vi "Initialize.vi"(7 "Serial Configuration":T1={"Baud Rate"=9600, "Flow Control"=0, "Parity"=0, "Data Bits"=8} {"Flow Control" items=["NONE", "SOFTWARE"]; "Data Bits" items=["7"=7, "8"=8]; "Parity" items=["NONE", "ODD", "EVEN"]; "Baud Rate" items=["300"=300, "600"=600, "1200"=1200, "2400"=2400, "4800"=4800, "9600"=9600, "19200"=19200]}, 8 "error in (no error)":errorcluster, 9 "Reset (True)":bool=TRUE, 10 "ID Query (True)":bool=TRUE, 11 "VISA resource name":refnum<visa-resource-name>) -> (0 "error out":errorcluster, 3 "VISA resource name out":refnum<visa-resource-name>)   [LabVIEW 2025, in "Chroma 19052.lvlib"]
doc: "Establishes communication with the instrument and optionally performs an instrument identification query and/or an instrument reset. It also places the instrument in a default state needed for other instrument driver operations. Therefore, call this VI before calling other instrument driver VIs for this instrument. Generally, you need to call the <b>Initialize</b> VI only once at the beginning of an application."
uses:
  <instrlib>/Chroma 19052/Chroma 19052.lvlib
  <vilib>/ErrorRing/Error Ring.xnode
panel:
  # "(c) 2025 RAMON TABOADA.  ALL RIGHTS RESERVED."
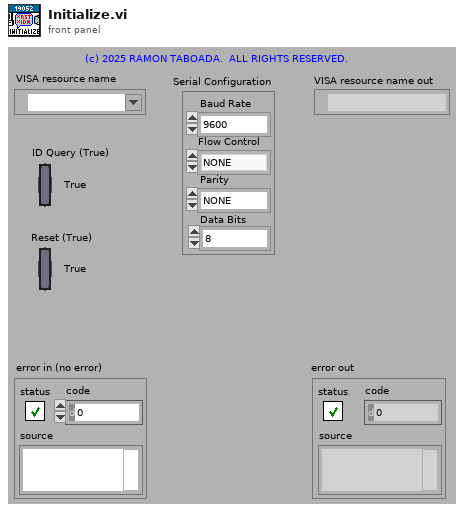
[diagram p1: front panel]
types:
  T1 = cluster{"Baud Rate":u32, "Flow Control":u16, "Parity":u16, "Data Bits":u16}
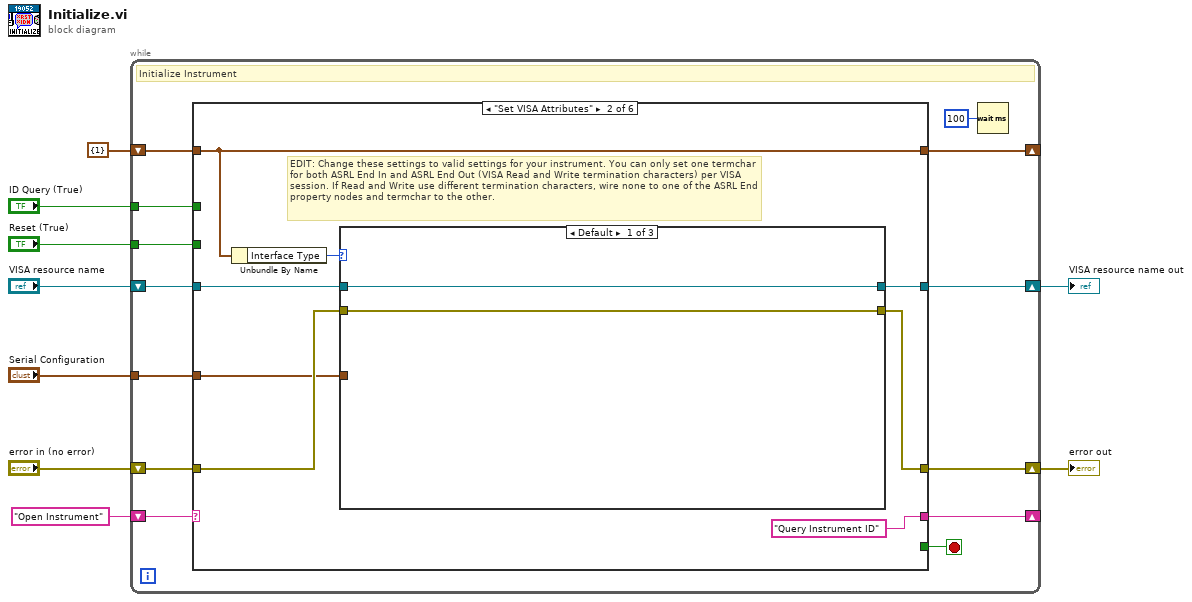
[diagram p0: block diagram]
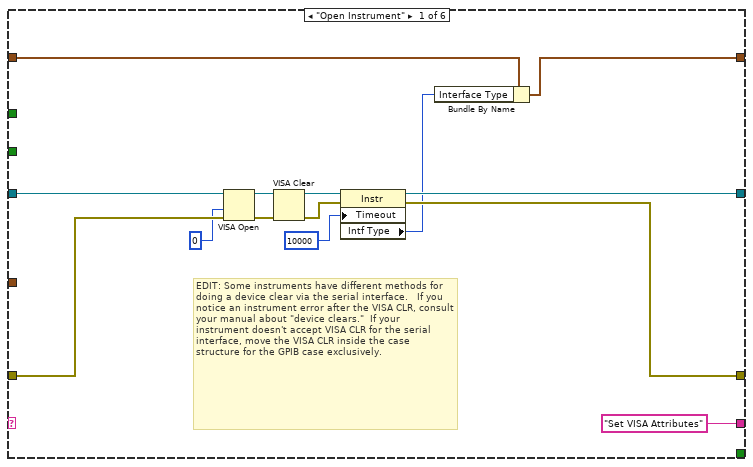
[diagram p2: hidden frame]
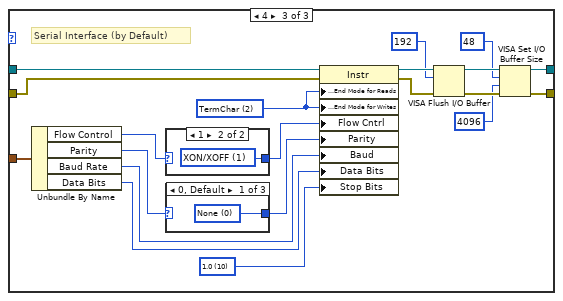
[diagram p4: hidden frame]
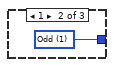
[diagram p5: hidden frame]
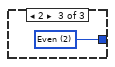
[diagram p6: hidden frame]
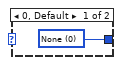
[diagram p7: hidden frame]
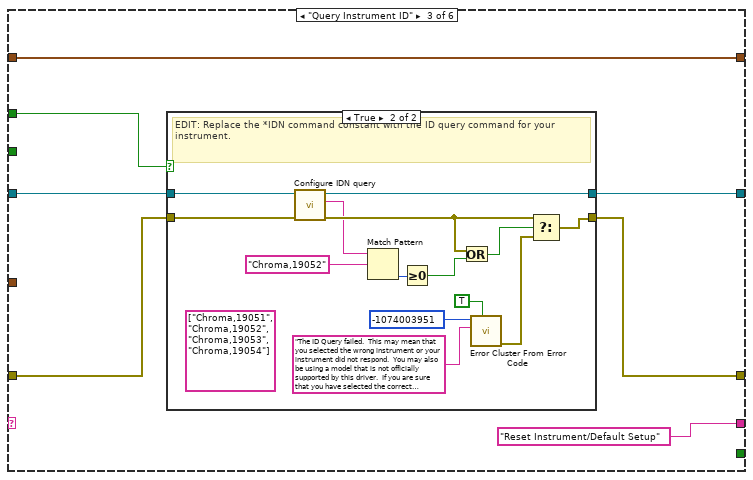
[diagram p8: hidden frame]
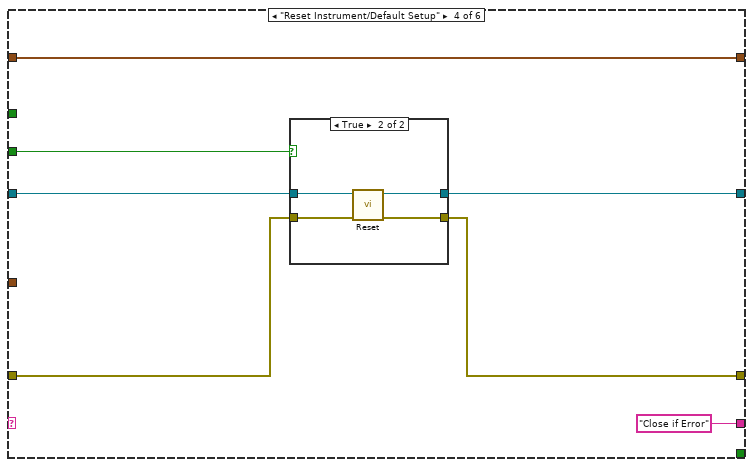
[diagram p10: hidden frame]
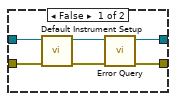
[diagram p11: hidden frame]
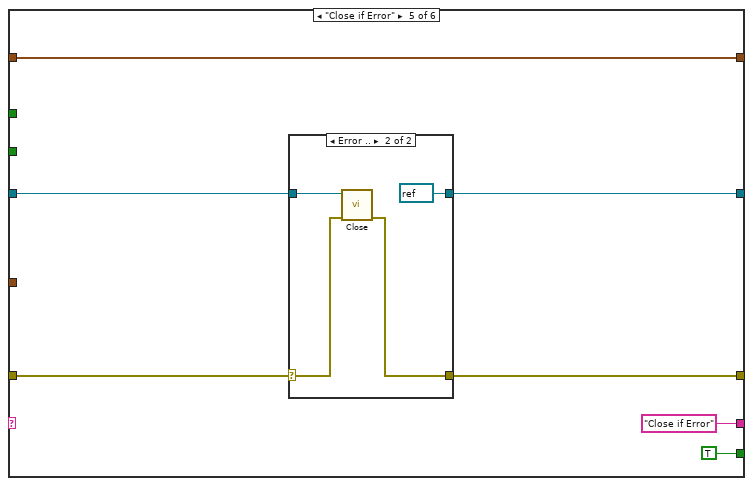
[diagram p12: hidden frame]
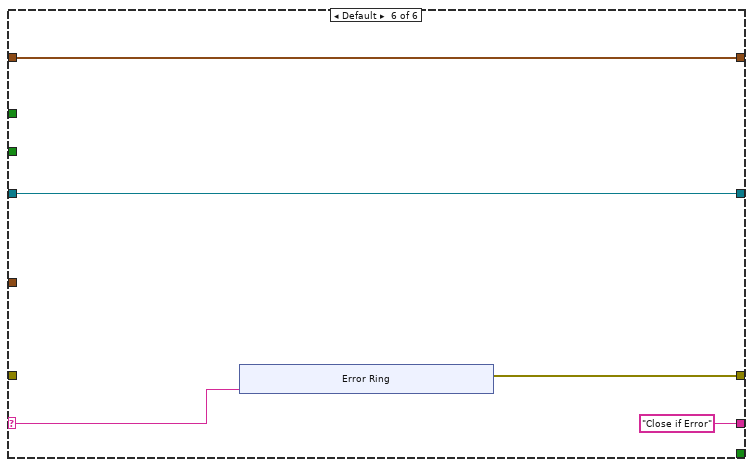
[diagram p14: hidden frame]
diagram:
  n1 = while {
    shift-right: [w21] -> _
    shift-left: cluster{"Interface Type":u16} {"Interface Type"=1} -> [w22]
    shift-right: [w20] -> _
    shift-left: "Open Instrument" -> [w11]
    tunnel: "Reset (True)" -> [w15]
    tunnel: "ID Query (True)" -> [w14]
    tunnel: "Serial Configuration" -> [w13]
    shift-right: [w18] -> w4
    shift-left: "VISA resource name" -> [w17]
    shift-right: [w19] -> w3
    shift-left: "error in (no error)" -> [w10]
    stop <- w16 stop-if-true
    # "Initialize Instrument"
    n2 = case shown="\"Set VISA Attributes\"" w11 {
      selector: w11 -> [_ _ _ _ _ w129]
      tunnel: w22 -> [w33 w44 w80 w103 w120 w131]
      tunnel: [w32 w44 w80 w103 w120 w131] -> w21
      tunnel: ["Set VISA Attributes" "Query Instrument ID" "Reset Instrument/Default Setup" "Close if Error" "Close if Error" "Close if Error"] -> w20
      tunnel: [w25 w37 w74 w97 w114 w128] -> w19
      tunnel: w10 -> [w34 w43 w78 w102 w117 _]
      tunnel: [w36 w42 w77 w100 w115 w130] -> w18
      tunnel: w17 -> [w29 w40 w79 w101 w116 w130]
      tunnel: [_ _ _ _ TRUE _] -> w16
      tunnel: w15 -> [_ _ _ w98 _ _]
      tunnel: w14 -> [_ _ w75 _ _ _]
      tunnel: w13 -> [_ w39 _ _ _ _]
      frame "Open Instrument" {
        # "EDIT: Some instruments have different methods for doing a device clear via the serial interface.   If you notice an instrument error after the VISA CLR, consult your manual about \"device clears.\"  If your instrument doesn't accept VISA CLR for the serial interface, move the VISA CLR inside the case  structure for the GPIB case exclusively."
        n3 = VISA Open(access mode=u32 0, error in (no error)=w34, VISA resource name=w29) -> (VISA resource name=w35:refnum<visa-resource-name>, error out=w30:errorcluster)  [unwired: 2 in]
        n4 = VISA Clear(VISA resource name=w35, error in (no error)=w30) -> (VISA resource name out=w28:refnum<visa-resource-name>, error out=w27:errorcluster)
        n5 = property class="Instr"(reference=w28, error in=w27, "Timeout"=u32 10000 ("Tmo Value")) -> (reference out=w36:refnum<visa-resource-name>, error out=w25:errorcluster, "Intf Type"=w23:u16)
        n6 = Bundle By Name(cluster=w33, "Interface Type"=w23) -> (w32:cluster{"Interface Type":u16})
      }
      frame "Set VISA Attributes" {
        # "EDIT: Change these settings to valid settings for your instrument. You can only set one termchar for both ASRL End In and ASRL End Out (VISA Read and Write termination characters) per VISA session. If Read and Write use different termination characters, wire none to one of the ASRL End property nodes and termchar to the other."
        n7 = Unbundle By Name(w44) -> ("Interface Type"=w38:u16)
        n8 = case shown="Default" w38 {
          tunnel: [w46 w47 w52] -> w42
          tunnel: [w45 w48 w54] -> w37
          tunnel: w43 -> [w45 w48 w67]
          tunnel: w40 -> [w46 w47 w68]
          tunnel: w39 -> [_ _ w57]
          frame Default {
          }
          frame 1 {
            # "GPIB when interface is installed"
          }
          frame 4 {
            w49 = u16 10 items=["1.0"=10, "1.5"=15, "2.0"=20] ("Serial Settings:Stop Bits")
            w65 = u16 2 items=["None", "LastBit", "TermChar"] ("Serial Settings:Serial End Mode for Reads")
            # "Serial Interface (by Default)"
            n9 = Unbundle By Name(w57) -> ("Flow Control"=w64:u16, "Parity"=w63:u16, "Baud Rate"=w61:u32, "Data Bits"=w60:u16)
            n10 = case shown="1" w64 {
              tunnel: [w72 w73] -> w59
              frame 0, Default {
                w72 = u16 0 items=["None", "XON/XOFF", "RTS/CTS", "XON/XOFF & RTS/CTS", "DTR/DSR", "XON/XOFF & DTR/DSR"] ("Serial Settings:Flow Control")
              }
              frame 1 {
                w73 = u16 1 items=["None", "XON/XOFF", "RTS/CTS", "XON/XOFF & RTS/CTS", "DTR/DSR", "XON/XOFF & DTR/DSR"] ("Serial Settings:Flow Control")
              }
            }
            n11 = case shown="0, Default" w63 {
              tunnel: [w69 w70 w71] -> w62
              frame 0, Default {
                w69 = u16 0 items=["None", "Odd", "Even", "Mark", "Space"] ("Serial Settings:Parity")
              }
              frame 1 {
                w70 = u16 1 items=["None", "Odd", "Even", "Mark", "Space"] ("Serial Settings:Parity")
              }
              frame 2 {
                w71 = u16 2 items=["None", "Odd", "Even", "Mark", "Space"] ("Serial Settings:Parity")
              }
            }
            n12 = property class="Instr"(reference=w68, error in=w67, "Serial Settings:End Mode for Reads"=w65, "Serial Settings:End Mode for Writes"=w65, "Flow Cntrl"=w59, "Parity"=w62, "Baud"=w61, "Data Bits"=w60, "Stop Bits"=w49) -> (reference out=w66:refnum<visa-resource-name>, error out=w58:errorcluster)
            n13 = VISA Flush I/O Buffer(VISA resource name=w66, mask (16)=u16 192, error in (no error)=w58) -> (VISA resource name out=w53:refnum<visa-resource-name>, error out=w55:errorcluster)
            n14 = VISA Set I/O Buffer Size(VISA resource name=w53, mask (16)=u16 48, size (4096)=u32 4096, error in (no error)=w55) -> (VISA resource name out=w52:refnum<visa-resource-name>, error out=w54:errorcluster)
          }
        }
      }
      frame "Query Instrument ID" {
        n15 = case shown="True" w75 {
          tunnel: [w81 w96] -> w74
          tunnel: [w82 w86] -> w77
          tunnel: w79 -> [w82 w90]
          tunnel: w78 -> [w81 w89]
          frame False {
          }
          frame True {
            (unwired) string[] ["Chroma,19051", "Chroma,19052", "Chroma,19053", "Chroma,19054"]
            # "EDIT: Replace the *IDN command constant with the ID query command for your instrument."
            n16 = call <instrlib>:"Configure IDN query.vi"("error in (no error)"=w89, "VISA resource name"=w90) -> ("error out"=w88:errorcluster, "Result"=w87:string, "VISA resource name out"=w86:refnum<visa-resource-name>)  [unwired: 7 in]
            n17 = Match Pattern(string=w87, regular expression="Chroma,19052") -> (offset past match=w85:i32)  [unwired: 1 in, 3 out]
            n18 = Greater Or Equal To 0?(x=w85) -> (x >= 0?=w83:bool)
            n19 = Or(x=w88, y=w83) -> (x .or. y?=w91:bool)
            n20 = call <vilib>:"Error Cluster From Error Code.vi"("show call chain? (False)"=TRUE, "error message (\"\")"="The ID Query failed.  This may mean that you selected the wrong instrument or your instrument did not respond.  You may also be using a model that is not officially supported by this driver.  If you are sure that you have selected the correct instrument and it is responding, try disabling the ID Query." ("Source (VI Name)"), "error code (0)"=-1074003951 ("Code")) -> ("error out"=w95:errorcluster)  [unwired: 6 in]
            n21 = Select(t=w88, s=w91, f=w95) -> (s? t:f=w96:errorcluster)
          }
        }
      }
      frame "Reset Instrument/Default Setup" {
        n22 = case shown="True" w98 {
          tunnel: w102 -> [w107 w113]
          tunnel: [w108 w112] -> w97
          tunnel: w101 -> [w105 w111]
          tunnel: [w109 w110] -> w100
          frame False {
            n23 = call <instrlib>:"Default Instrument Setup.vi"("error in (no error)"=w107, "VISA resource name"=w105) -> ("error out"=w106:errorcluster, "VISA resource name out"=w104:refnum<visa-resource-name>)  [unwired: 8 in]
            n24 = call <instrlib>:"Error Query.vi"("error in (no error)"=w106, "VISA resource name"=w104) -> ("error out"=w108:errorcluster, "VISA resource name out"=w109:refnum<visa-resource-name>)  [unwired: 6 in, 2 out]
          }
          frame True {
            n25 = call <instrlib>:"Reset.vi"("error in (no error)"=w113, "VISA resource name"=w111) -> ("error out"=w112:errorcluster, "VISA resource name out"=w110:refnum<visa-resource-name>)  [unwired: 8 in]
          }
        }
      }
      frame "Close if Error" {
        n26 = case shown="Error .." w117 {
          selector: w117 -> [w122 w125]
          tunnel: w116 -> [w121 w123]
          tunnel: [w121 refnum<visa-resource-name> refnum ("VISA resource name")] -> w115
          tunnel: [w122 w124] -> w114
          frame No Error {
          }
          frame Error {
            n27 = call <instrlib>:"Close.vi"("error in (no error)"=w125, "VISA resource name"=w123) -> ("error out"=w124:errorcluster)  [unwired: 9 in]
          }
        }
      }
      frame Default {
        n28 = xnode "Error Ring"("parameter 0"=w129) -> ("error out"=w128:errorcluster)
      }
    }
    n29 = Wait (ms)(milliseconds to wait=u32 100) -> ()  [unwired: 1 out]
  }
  "VISA resource name out" <- w4
  "error out" <- w3
